vi "String is a number.vi"(11 "Baud Rate":string) -> (3 "Boolean":bool)   [LabVIEW 2020, in "Modbus Master System Explorer.lvlib"]
uses:
  Modbus Master System Explorer.lvlib
  <vilib>/regexp/Match Regular Expression.xnode
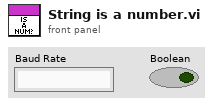
[diagram p1: front panel]
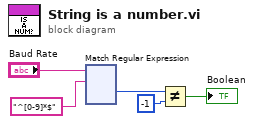
[diagram p0: block diagram]
diagram:
  n1 = xnode "Match Regular Expression"("input string"="Baud Rate", "regular expression"="^[0-9]*$") -> ("offset past match"=w3:i32)  [unwired: 4 in, 4 out]
  n2 = Not Equal?(x=w3, y=-1) -> (x != y?=→"Boolean":bool)
